vi "遥控手柄.vi"() -> (0 "error out":errorcluster, 1 "显示界面":T1, 2 "device ID":refnum<k1>)   [LabVIEW 2018]
uses:
  <vilib>/Utility/inputDevices.llb/joystickAcquire.vi
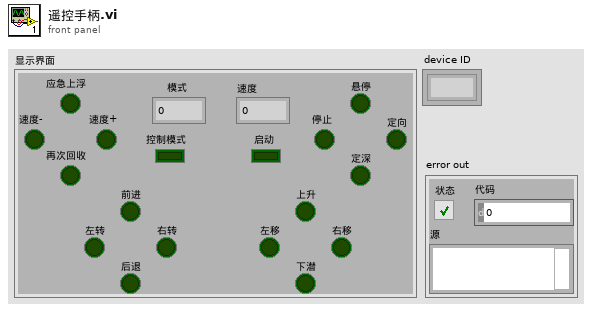
[diagram p1: front panel]
types:
  T1 = cluster{"右转":bool, "左转":bool, "后退":bool, "前进":bool, "右移":bool, "左移":bool, "下潜":bool, "上升":bool, "定深":bool, "定向":bool, "停止":bool, "悬停":bool, "控制模式":bool, "启动":bool, "应急上浮":bool, "再次回收":bool, "速度+":bool, "速度-":bool, "模式":i32, "速度":i32}
  T2 = cluster{"X axis":i32, "Y axis":i32, "Z axis":i32, "X axis rotation":i32, "Y axis rotation":i32, "Z axis rotation":i32, "U axis":i32, "V axis":i32}
  T3 = cluster{"button 1":bool, "button 2":bool, "button 3":bool, "button 4":bool, "button 5":bool, "button 6":bool, "button 7":bool, "button 8":bool, "button 9":bool, "button 10":bool, "button 11":bool, "button 12":bool, "button 13":bool, "button 14":bool, "button 15":bool, "button 16":bool, "button 17":bool, "button 18":bool, "button 19":bool, "button 20":bool, "button 21":bool, "button 22":bool, "button 23":bool, "button 24":bool, "button 25":bool, "button 26":bool, "button 27":bool, "button 28":bool, "button 29":bool, "button 30":bool, "button 31":bool, "button 32":bool}
  T4 = cluster{"pov 1":i32, "pov 2":i32, "pov 3":i32, "pov 4":i32}
  T5 = cluster{bool, bool, bool, bool, bool, bool, bool, bool, "Value":bool, "Value":bool, "button 3":bool, "Value":bool, "button 7":bool, "button 8":bool, bool, bool, bool, bool, "x":i32, "上限":i32}
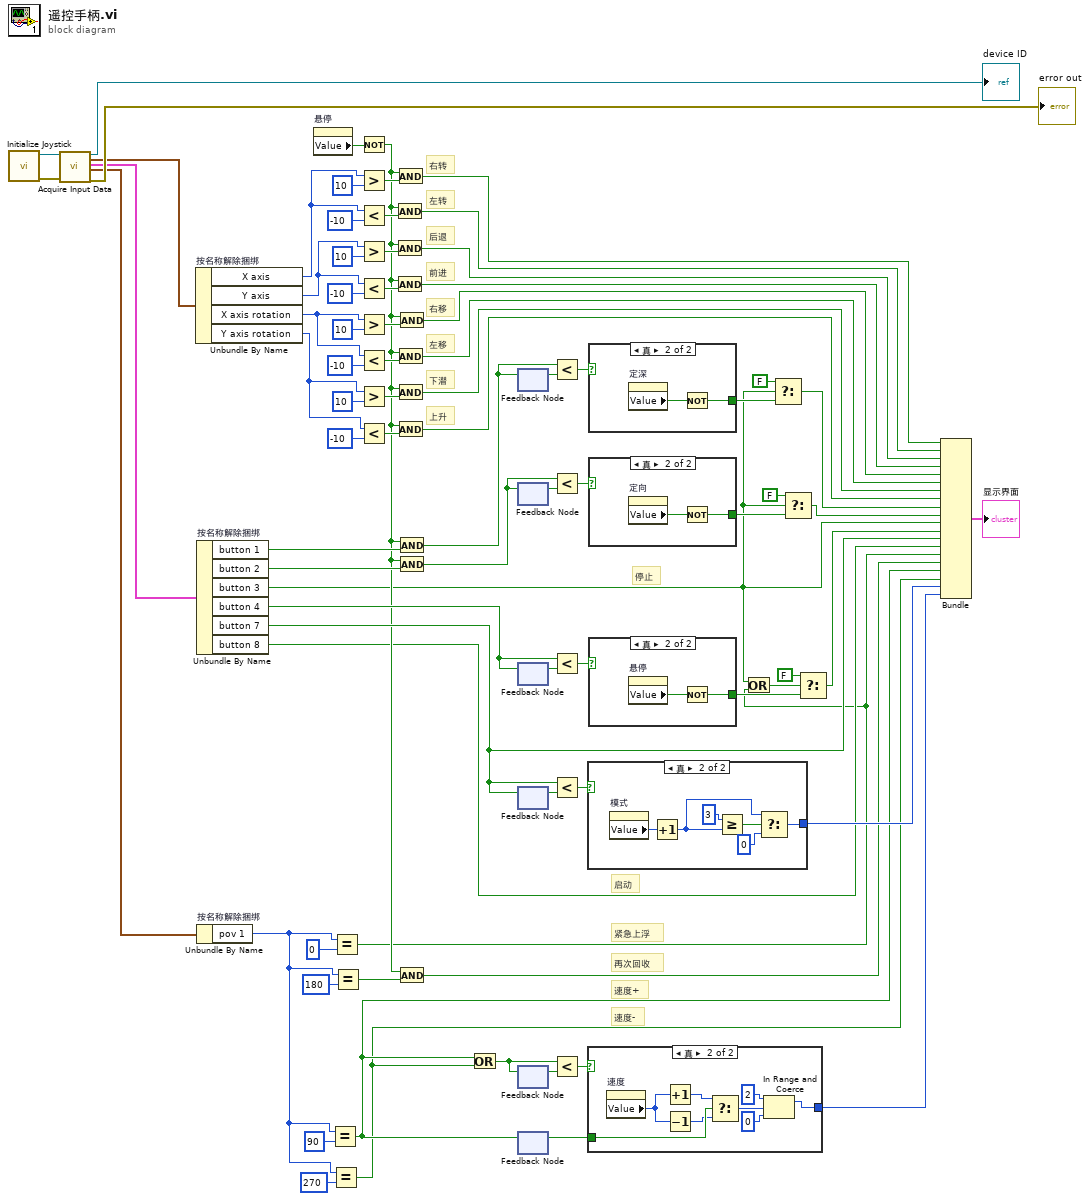
[diagram p0: block diagram]
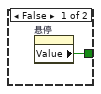
[diagram p2: hidden frame]
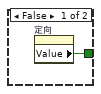
[diagram p3: hidden frame]
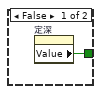
[diagram p4: hidden frame]
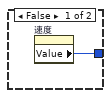
[diagram p5: hidden frame]
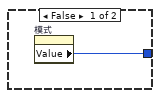
[diagram p6: hidden frame]
diagram:
  # "上升"
  # "下潜"
  # "左移"
  # "右移"
  # "前进"
  # "后退"
  # "左转"
  # "右转"
  # "速度-"
  # "速度+"
  # "再次回收"
  # "紧急上浮"
  # "启动"
  # "停止"
  n1 = call <vilib>:"Initialize Joystick.vi"() -> ("error out"=w74:errorcluster, "device ID"=w78:refnum<k1>)  [unwired: 10 in]
  n2 = call-poly <vilib>:"Acquire Input Data.vi"("device ID"=w78, "error in (no error)"=w74) -> ("device ID"=→"device ID":refnum<k1>, "axis info"=w77:T2, "button info"=w76:T3, "direction info"=w75:T4, "error out"=→"error out":errorcluster)  [unwired: 13 in]
  n3 = Unbundle By Name "按名称解除捆绑"(w77) -> ("X axis"=w72:i32, "Y axis"=w68:i32, "X axis rotation"=w65:i32, "Y axis rotation"=w62:i32)
  n4 = Unbundle By Name "按名称解除捆绑"(w76) -> ("button 1"=w20:bool, "button 2"=w18:bool, "button 3"=w1:bool, "button 4"=w50:bool, "button 7"=w21:bool, "button 8"=w13:bool)
  n5 = Unbundle By Name "按名称解除捆绑"(w75) -> ("pov 1"=w57:i32)
  n6 = property on="悬停" class="Bool (严格)"() -> ("Value"=w41:bool)  [unwired: 2 in, 2 out]
  n7 = Equal?(x=w57, y=90) -> (x = y?=w23:bool)
  n8 = Equal?(x=w57, y=270) -> (x = y?=w22:bool)
  n9 = Equal?(x=w57, y=0) -> (x = y?=w9:bool)
  n10 = Equal?(x=w57, y=180) -> (x = y?=w16:bool)
  n11 = Not(x=w41) -> (.not. x?=w14:bool)
  n12 = Greater?(x=w72, y=10) -> (0:w39:bool)
  n13 = Less?(x=w72, y=-10) -> (x < y?=w37:bool)
  n14 = Greater?(x=w68, y=10) -> (0:w35:bool)
  n15 = Less?(x=w68, y=-10) -> (x < y?=w33:bool)
  n16 = Greater?(x=w65, y=10) -> (0:w31:bool)
  n17 = Less?(x=w65, y=-10) -> (x < y?=w30:bool)
  n18 = Greater?(x=w62, y=10) -> (0:w27:bool)
  n19 = Less?(x=w62, y=-10) -> (x < y?=w25:bool)
  n20 = And(x=w14, y=w37) -> (x .and. y?=w38:bool)
  n21 = And(x=w14, y=w35) -> (x .and. y?=w36:bool)
  n22 = And(x=w14, y=w33) -> (x .and. y?=w34:bool)
  n23 = And(x=w14, y=w39) -> (x .and. y?=w40:bool)
  n24 = And(x=w14, y=w30) -> (x .and. y?=w29:bool)
  n25 = And(x=w14, y=w27) -> (x .and. y?=w28:bool)
  n26 = And(x=w14, y=w25) -> (x .and. y?=w26:bool)
  n27 = And(x=w14, y=w31) -> (x .and. y?=w32:bool)
  n28 = And(x=w14, y=w20) -> (x .and. y?=w19:bool)
  n29 = And(x=w14, y=w18) -> (x .and. y?=w17:bool)
  n30 = And(x=w14, y=w16) -> (x .and. y?=w15:bool)
  n31 = Or(x=w23, y=w22) -> (x .or. y?=w47:bool)
  n32 = feedback #1() -> (w56:bool)  [unwired: 1 in]
  n33 = feedback-in #1(w19) -> ()
  n34 = feedback #2() -> (w52:bool)  [unwired: 1 in]
  n35 = feedback-in #2(w17) -> ()
  n36 = feedback #3() -> (w51:bool)  [unwired: 1 in]
  n37 = feedback-in #3(w50) -> ()
  n38 = feedback #4() -> (w46:bool)  [unwired: 1 in]
  n39 = feedback-in #4(w21) -> ()
  n40 = feedback #5() -> (w48:bool)  [unwired: 1 in]
  n41 = feedback-in #5(w47) -> ()
  n42 = feedback #6() -> (w42:bool)  [unwired: 1 in]
  n43 = feedback-in #6(w23) -> ()
  n44 = Less?(x=w19, y=w56) -> (x < y?=w55:bool)
  n45 = Less?(x=w17, y=w52) -> (x < y?=w54:bool)
  n46 = Less?(x=w50, y=w51) -> (x < y?=w53:bool)
  n47 = Less?(x=w21, y=w46) -> (x < y?=w24:bool)
  n48 = Less?(x=w47, y=w48) -> (x < y?=w43:bool)
  n49 = case shown="真" w24 {
    tunnel: [w81 w84] -> w45
    frame False {
      n50 = property on="模式" class="DigNum (严格)"() -> ("Value"=w81:i32)  [unwired: 2 in, 2 out]
    }
    frame True {
      n51 = property on="模式" class="DigNum (严格)"() -> ("Value"=w83:i32)  [unwired: 2 in, 2 out]
      n52 = Increment(x=w83) -> (x+1=w82:i32)
      n53 = Greater Or Equal?(x=3, y=w82) -> (x >= y?=w86:bool)
      n54 = Select(t=w82, s=w86, f=0 ("x")) -> (s? t:f=w84:i32)
    }
  }
  n55 = case shown="真" w43 {
    tunnel: [w88 w92] -> w44
    tunnel: w42 -> [_ w96]
    frame False {
      n56 = property on="速度" class="DigNum (严格)"() -> ("Value"=w88:i32)  [unwired: 2 in, 2 out]
    }
    frame True {
      n57 = property on="速度" class="DigNum (严格)"() -> ("Value"=w90:i32)  [unwired: 2 in, 2 out]
      n58 = Increment(x=w90) -> (x+1=w91:i32)
      n59 = Decrement(x=w90) -> (x-1=w89:i32)
      n60 = Select(t=w91, s=w96, f=w89) -> (s? t:f=w95:i32)
      n61 = In Range and Coerce(upper limit=2 ("上限"), x=w95, lower limit=0 ("下限")) -> (coerced(x)=w92:i32)  [unwired: 1 out]
    }
  }
  n62 = case shown="真" w55 {
    tunnel: [w97 w98] -> w3
    frame False {
      n63 = property on="定深" class="Bool (严格)"() -> ("Value"=w97:bool)  [unwired: 2 in, 2 out]
    }
    frame True {
      n64 = property on="定深" class="Bool (严格)"() -> ("Value"=w99:bool)  [unwired: 2 in, 2 out]
      n65 = Not(x=w99) -> (.not. x?=w98:bool)
    }
  }
  n66 = case shown="真" w54 {
    tunnel: [w100 w101] -> w6
    frame False {
      n67 = property on="定向" class="Bool (严格)"() -> ("Value"=w100:bool)  [unwired: 2 in, 2 out]
    }
    frame True {
      n68 = property on="定向" class="Bool (严格)"() -> ("Value"=w102:bool)  [unwired: 2 in, 2 out]
      n69 = Not(x=w102) -> (.not. x?=w101:bool)
    }
  }
  n70 = case shown="真" w53 {
    tunnel: [w103 w104] -> w10
    frame False {
      n71 = property on="悬停" class="Bool (严格)"() -> ("Value"=w103:bool)  [unwired: 2 in, 2 out]
    }
    frame True {
      n72 = property on="悬停" class="Bool (严格)"() -> ("Value"=w105:bool)  [unwired: 2 in, 2 out]
      n73 = Not(x=w105) -> (.not. x?=w104:bool)
    }
  }
  n74 = Or(x=w1, y=w9) -> (x .or. y?=w8:bool)
  n75 = Select(t=FALSE ("f"), s=w1, f=w3) -> (s? t:f=w2:bool)
  n76 = Select(t=FALSE ("f"), s=w1, f=w6) -> (s? t:f=w5:bool)
  n77 = Select(t=FALSE ("f"), s=w8, f=w10) -> (s? t:f=w12:bool)
  n78 = Bundle(w40, w38, w36, w34, w32, w29, w28, w26, "Value"=w2, "Value"=w5, "button 3"=w1, "Value"=w12, "button 7"=w21, "button 8"=w13, w9, w15, w23, w22, "x"=w45, "上限"=w44) -> (→"显示界面":T5)  [unwired: 1 in]
